vi "Error.Remove Trace Info form Error Desc.vi"(7 "Logging Level":T1, 10 "error in":errorcluster, 11 "Leave In Trace Info":bool) -> (2 "error out":errorcluster)   [LabVIEW 2024, in "EQMF.lvlib" / "Errors.lvlib"]
uses:
  <vilib>/KATE/Event Log/Event Notification/Event Log.Log Level.ctl
  <vilib>/Utility/error.llb/Trim Whitespace One-Sided.vi
  Errors.lvlib
  <vilib>/KATE/Event Log/Event Log.lvlib
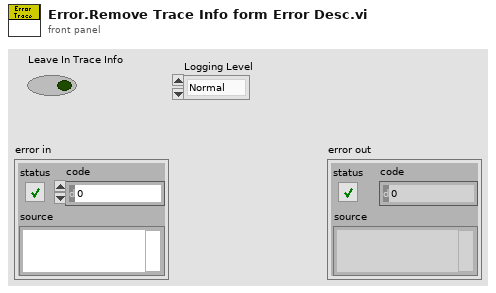
[diagram p1: front panel]
types:
  T1 = typedef "KATE_Lib.lvlib/Event Log.lvlib/Event Log.Log Level.ctl" = enum16{"Normal", "Verbose", "Debug0", "Debug1", "Debug2"}
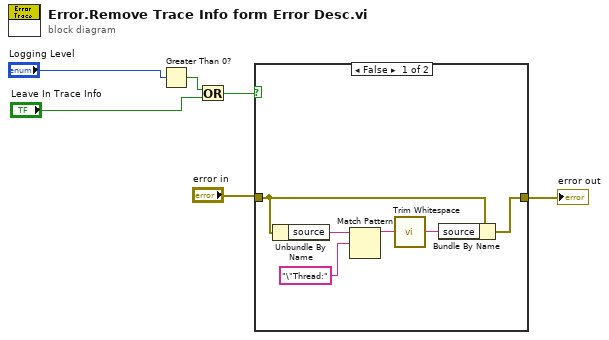
[diagram p0: block diagram]
diagram:
  n1 = Greater Than 0?(x="Logging Level") -> (x > 0?=w4:bool)
  n2 = Or(x=w4, y="Leave In Trace Info") -> (x .or. y?=w1:bool)
  n3 = case shown="False" w1 {
    tunnel: "error in" -> [w9 w13]
    tunnel: [w8 w13] -> w5
    frame False {
      n4 = Unbundle By Name(w9) -> ("source"=w12:string)
      n5 = Match Pattern(string=w12, regular expression="\"Thread:") -> (before substring=w10:string)  [unwired: 1 in, 3 out]
      n6 = call <vilib>:"Trim Whitespace.vi"("string"=w10) -> ("trimmed string"=w7:string)  [unwired: 1 in]
      n7 = Bundle By Name(cluster=w9, "source"=w7) -> (w8:errorcluster)
    }
    frame True {
    }
  }
  "error out" <- w5
